vi "Get Project Items.vi"(8 "error in (no error)":errorcluster, 10 "type":string, 11 "project in":refnum<vi>) -> (0 "error out":errorcluster, 2 "project items":refnum<vi>[](array[refnum]), 3 "project out":refnum<vi>)   [LabVIEW 2017]
doc: "Returns <b>project in</b> items references.\n\nMost common types are: VI, Library, LVLibp, LVClass, Class Private Data, XControl, Ability VI, Folder, Document."
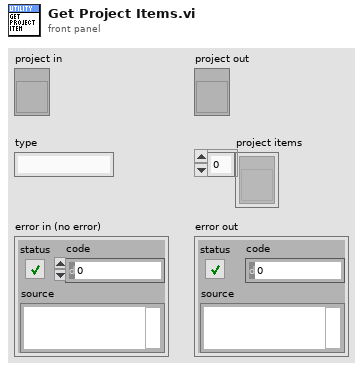
[diagram p1: front panel]
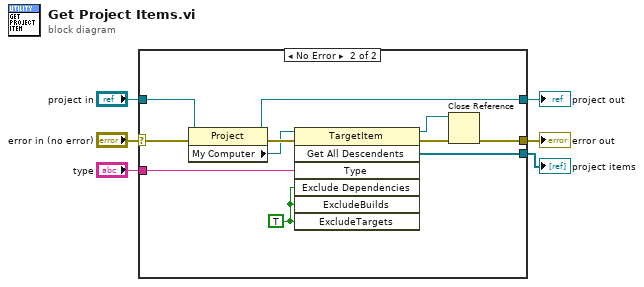
[diagram p0: block diagram]
diagram:
  n1 = case shown="No Error" "error in (no error)" {
    selector: "error in (no error)" -> [w8 w10]
    tunnel: "project in" -> [w7 w19]
    tunnel: [w7 w18] -> w5
    tunnel: [_ w15] -> w4
    tunnel: [w8 w11] -> w2
    tunnel: "type" -> [_ w9]
    frame Error {
    }
    frame No Error {
      w12 = TRUE ("ExcludeTargets")
      n2 = property class="Project"(reference=w19, error in=w10) -> (reference out=w18:refnum<vi>, error out=w16:errorcluster, "My Computer"=w14:refnum<vi>)
      n3 = invoke class="TargetItem" method="Get All Descendents"(reference=w14, error in=w16, "Type"=w9, "Exclude Dependencies"=w12, "ExcludeBuilds"=w12, "ExcludeTargets"=w12) -> (reference out=w13:refnum<vi>, error out=w17:errorcluster, "All Descendents"=w15:refnum<vi>[])  [unwired: 1 in, 4 out]
      n4 = Close Reference(reference=w13, error in (no error)=w17) -> (error out=w11:errorcluster)
    }
  }
  "project out" <- w5
  "project items" <- w4
  "error out" <- w2
